vi "20newsgroups_vectorized.vi"(8 "error in (no error)":errorcluster caption="entrée d'erreur (pas d'erreur)", 11 "fetch_20newsgroups_vectorized":T1={"subset"="train", "remove"=[], "download_if_missing"=TRUE, "normalize"=TRUE, "Returns"="Data"}) -> (0 "error out":errorcluster, 3 "Data":T2)   [LabVIEW 2020]
doc: "Load the 20 newsgroups dataset and vectorize it into token counts (classification).\n\nData Set Characteristics : \n - Classes : 20\n - Samples total : 18846\n - Dimensionality : 130107\n - Features : real\n\nParameters : \n\n- subset : ‘train’ or ‘test’, ‘all’, optional\nSelect the dataset to load: ‘train’ for the training set, ‘test’ for the test set, ‘all’ for both, with shuffled ordering.\n\n- remove : tuple\nMay contain any subset of (‘headers’, ‘footers’, ‘quotes’). Each of these are kinds of text that will be detected and removed from the newsgroup posts, preventing classifiers from overfitting on metadata.\n\n‘headers’ removes newsgroup headers, ‘footers’ removes blocks at the ends of posts that look like signatures, and ‘quotes’ removes lines that appear to be quoting another post.\n\n- download_if_missing : optional, True by default\nIf False, raise an IOError if the data is not locally available instead of trying to download the data from the source site.\n\nnormalize : bool, default=True\nIf True, normalizes each document’s feature vector to unit norm using sklearn.preprocessing.normalize.\n\n\nReturns :\n\n- data : sparse matrix, shape [n_samples, n_features]\n The data matrix to learn.\n\n- target : array, shape [n_samples]\n The target labels."
uses:
  20newsgroups_vectorized.lvclass
panel:
  out "20newsgroups_vectorized.lvclass":refnum<class "20newsgroups_vectorized.lvclass">
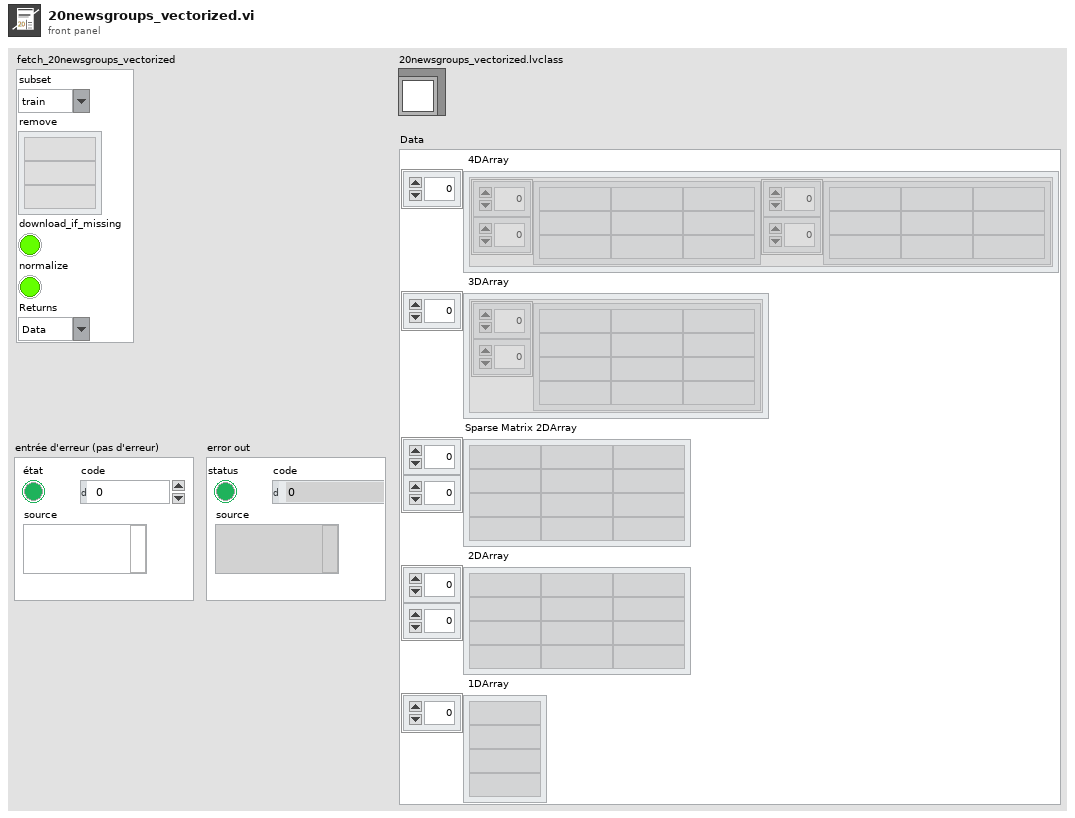
[diagram p1: front panel]
types:
  T1 = cluster{"subset":string, "remove":string[], "download_if_missing":bool, "normalize":bool, "Returns":string}
  T2 = cluster{" 4DArray":cluster{"1":string[][], "2":string[][]}[], " 3DArray":cluster{"Tableau":string[][]}[], "Sparse Matrix 2DArray":string[][], " 2DArray":string[][], " 1DArray":string[]}
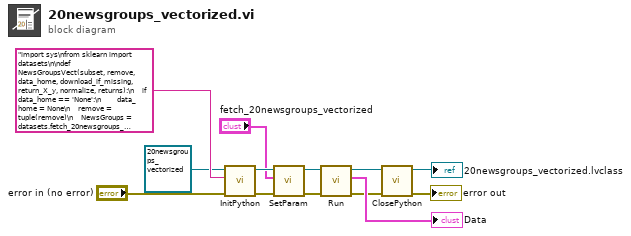
[diagram p0: block diagram]
diagram:
  n1 = call-dynamic "InitPython.vi"("error in (no error)"="error in (no error)", "Python Instruction"="import sys\nfrom sklearn import datasets\n\ndef NewsGroupsVect(subset, remove, data_home, download_if_missing, return_X_y, normalize, returns):\n    if data_home == 'None':\n        data_home = None\n    remove = tuple(remove)\n    NewsGroups = datasets.fetch_20newsgroups_vectorized(subset, remove, data_home, download_if_missing, return_X_y, normalize)\n    try:\n        if returns == 'Data' :\n            data = NewsGroups['data']\n            Mat = data.tocoo()\n            return str(list(zip(Mat.row, Mat.col, Mat.data)))\n        else :\n            data = NewsGroups['target'].tolist()\n            return str(data)\n    except:\n        erreur = sys.exc_info()\n        typerr = u\"%s\" % (erreur[0])\n        typerr = typerr[typerr.find(\"'\")+1:typerr.rfind(\"'\")]\n        msgerr = u\"%s\" % (erreur[1])\n        message = str('/!\\\\ {0} : {1}'. format(typerr,msgerr))\n        return message", "Scikit-learn en entrée"=refnum<class "20newsgroups_vectorized.lvclass"> refnum ("20newsgroups_vectorized.lvclass")) -> ("error out"=w9:errorcluster, "Scikit-learn en sortie"=w10:refnum<class "20newsgroups_vectorized.lvclass">)  [unwired: 7 in]
  n2 = call-dynamic "SetParam.vi"("error in (no error)"=w9, "fetch_20newsgroups_vectorized"="fetch_20newsgroups_vectorized", "20newsgroups_vectorized.lvclass"=w10) -> ("error out"=w6:errorcluster, "20newsgroups_vectorized.lvclass"=w7:refnum<class "20newsgroups_vectorized.lvclass">)  [unwired: 7 in]
  n3 = call-dynamic "Run.vi"("error in (no error)"=w6, "20newsgroups_vectorized.lvclass"=w7) -> ("error out"=w2:errorcluster, "Data"=→"Data":T2, "20newsgroups_vectorized.lvclass 2"=w3:refnum<class "20newsgroups_vectorized.lvclass">)  [unwired: 7 in]
  n4 = call-dynamic "ClosePython.vi"("error in (no error)"=w2, "Scikit-learn en entrée"=w3) -> ("error out"=→"error out":errorcluster, "Scikit-learn en sortie"=→"20newsgroups_vectorized.lvclass":refnum<class "20newsgroups_vectorized.lvclass">)  [unwired: 8 in]
